vi "Find Max Constant.vi"(1 "constants":cluster{"a":dbl, "b":dbl, "c":dbl, "d":dbl}) -> (0 "Max or 1":dbl)   [LabVIEW 2016]
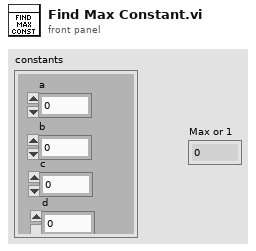
[diagram p1: front panel]
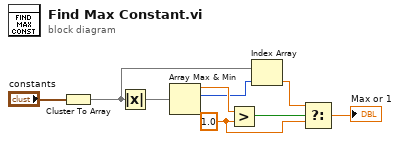
[diagram p0: block diagram]
diagram:
  w6 = 1.0 ("y")
  n1 = Cluster To Array(cluster="constants") -> (array=w2:dbl[])
  n2 = Absolute Value(x=w2) -> (abs(x)=w4:dbl[])
  n3 = Array Max & Min(array=w4) -> (max value=w7:dbl, max index (indices)=w1:i32)  [unwired: 2 out]
  n4 = Greater?(x=w7, y=w6) -> (0:w8:bool)
  n5 = Index Array(array=w2, index=w1) -> (element=w3:dbl)
  n6 = Select(t=w3, s=w8, f=w6) -> (s? t:f=→"Max or 1":dbl)
